vi "PPFS_Robot Main.vi"   [LabVIEW 2019]
doc: "This VI implements the framework and scheduler for your robotics program. It should not be necessary to modify the framework. You are expected to add your code to the VIs called from Robot Main - the ones located in the Team Code folder within the project."
panel:
  # "Execution notes:\n - Copy the file default_navgrid.json from the deploy\n    directory in this project to %USERPROFILE%\\\n    Documents\\LabVIEW Data\\ directory \n - Start driver station before running this VI"
types:
  T1 = enum32{"Invalid", "Standard", "Closed", "Hidden", "Minimized", "Maximized"}
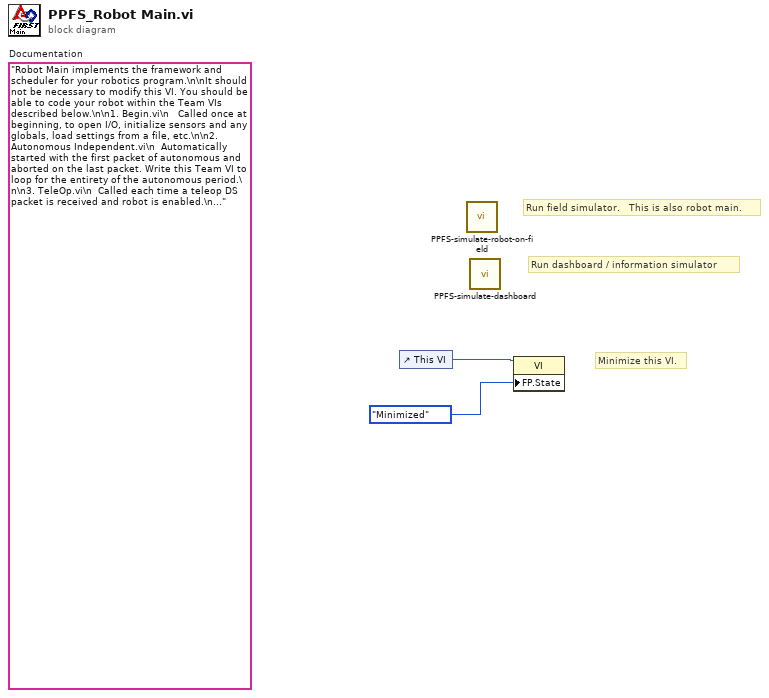
[diagram p0: block diagram]
diagram:
  (unwired) "Robot Main implements the framework and scheduler for your robotics program.\n\nIt should not be necessary to modify this VI. You should be able to code your robot within the Team VIs described below.\n\n1. Begin.vi\n   Called once at beginning, to open I/O, initialize sensors and any globals, load settings from a file, etc.\n\n2. Autonomous Independent.vi\n  Automatically started with the first packet of autonomous and aborted on the last packet. Write this Team VI to loop for the entirety of the autonomous period.\n\n3. TeleOp.vi\n  Called each time a teleop DS packet is received and robot is enabled.\n\n4. Disabled.vi\n  Called each time a packet is received and the robot is disabled.\n\n5. Test.vi\n  Called Automatically started with the first test packet and aborted on the last. Modify this VI to carry out robot and sensor validation tests.\n\n6. Vision Processing.vi\n  A parallel loop that acquires and processes camera images. Drag from the project/Team Code if you wish to use this.\n\n7. PeriodicTasks.vi\n  Parallel loops running at user-defined rates.\n\n8. Finish.vi\n  Called before exiting, so you can save data, clean up I/O, etc.\n"  # Documentation
  # "Minimize this VI."
  # "Run dashboard / information simulator"
  # "Run field simulator.   This is also robot main."
  n1 = control-ref of="This VI"() -> (w2:refnum<vi>)
  n2 = call "PPFS-simulate-robot-on-field.vi"() -> ()  [unwired: 12 in]
  n3 = call "PPFS-simulate-dashboard.vi"() -> ()  [unwired: 12 in]
  n4 = property class="VI"(reference=w2, "FP.State"=T1."Minimized" ("Front Panel Window:State")) -> ()  [unwired: 1 in, 2 out]
